vi "Close.vi"(8 "Error In":errorcluster) -> (0 "Error Out":errorcluster)   [LabVIEW 2018, in "Database.lvlib"]
uses:
  Database.lvlib
  Action.ctl
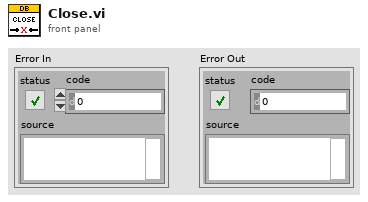
[diagram p1: front panel]
types:
  T1 = typedef "Database.lvlib/Action.ctl" = enum16{"Init", "List Tables", "List Columns", "Query", "Close"}
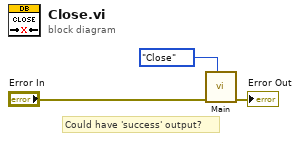
[diagram p0: block diagram]
diagram:
  # "Could have 'success' output?"
  n1 = call "Main.vi"("Action"=Action."Close", "Error In"="Error In") -> ("Error Out"=→"Error Out":errorcluster)  [unwired: 8 in, 1 out]
